vi "test.vi"() -> ()   [LabVIEW 2012]
panel:
  in  "y_start":u32=1
  in  "x_start":u32=1
  in  "ImageCnt":u32=1
  out "ImageCnt":u32
  out "y_end":u32
  out "y_start":u32
  out "x_end":u32
  out "x_start":u32
  out "强度图":i16[][](graph)
  in  "sim":bool
  in  "path":path
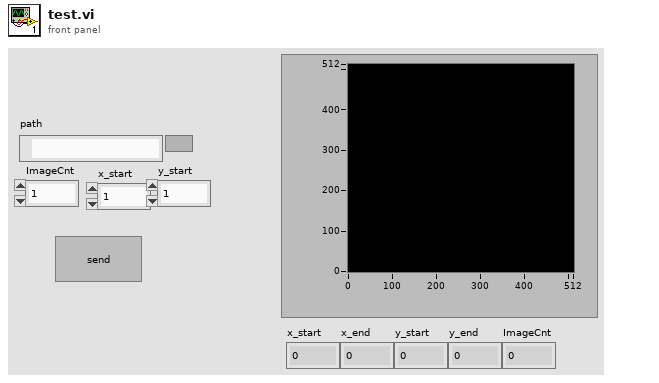
[diagram p1: front panel]
types:
  T1 = cluster{"image":i16[][], "x_start":u32, "x_end":u32, "y_start":u32, "y_end":u32, "ImageCnt":u32}
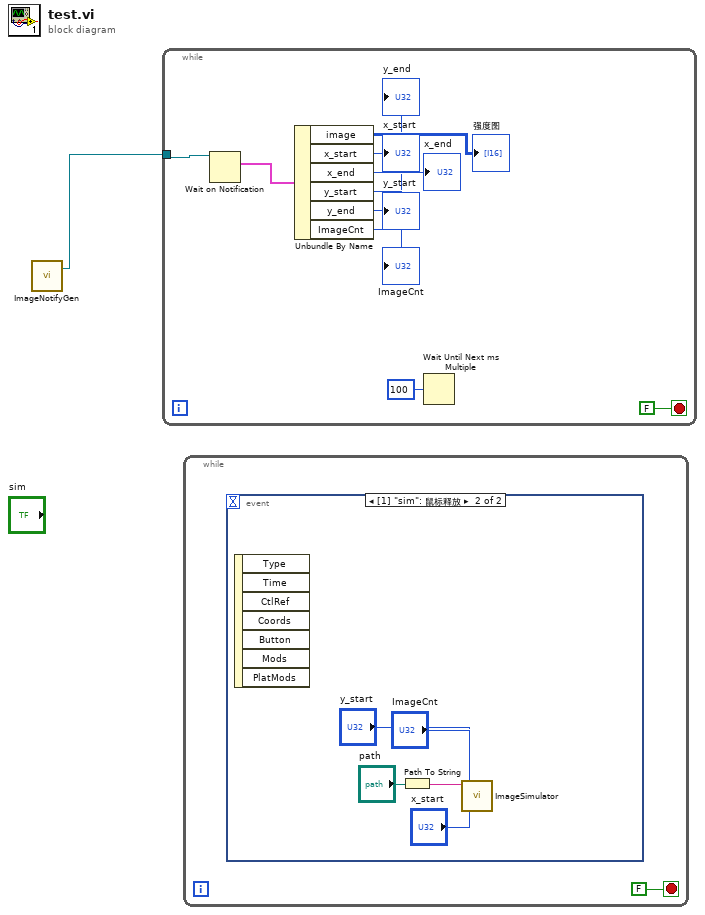
[diagram p0: block diagram]
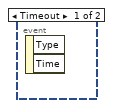
[diagram p2: hidden frame]
diagram:
  n1 = call "ImageNotifyGen.vi"() -> ("ImageNotify"=w1:refnum<notifier>)  [unwired: 2 in, 1 out]
  n2 = while {
    tunnel: w1 -> [w3]
    stop <- FALSE stop-if-true
    n3 = Wait on Notification(notifier=w3) -> (notification=w2:T1)  [unwired: 3 in, 3 out]
    n4 = Unbundle By Name(w2) -> ("image"=→"强度图":i16[][], "x_start"=→"x_start":u32, "x_end"=→"x_end":u32, "y_start"=→"y_start":u32, "y_end"=→"y_end":u32, "ImageCnt"=→"ImageCnt":u32)
    n5 = Wait Until Next ms Multiple(millisecond multiple=u32 100 ("毫秒倍数")) -> ()  [unwired: 1 out]
  }
  n6 = while {
    stop <- FALSE stop-if-true
    n7 = event shown="[1] \"sim\": 鼠标释放" {
      selector: _ -> [_ _]
      dyn-events: _ -> [_ _]
      timeout: _ -> [_ _]
      event Timeout {
        n8 = event-data() -> ()  [unwired: 1 in, 2 out]
      }
      event "sim": Mouse Up {
        n9 = event-data() -> ()  [unwired: 1 in, 7 out]
        n10 = Path To String(path="path") -> (string=w16:string)
        n11 = call "ImageSimulator.vi"("y_start"="y_start", "x_start"="x_start", "ImageCnt"="ImageCnt", "FilePath"=w16) -> ()  [unwired: 1 in]
      }
    }
  }
